vi "Query Deviation.vi"(8 "error in (no error)":errorcluster, 10 "Deviation Mode (0: Reading)":u16(ring) items=["Reading", "Absolute"], 11 "VISA resource name":refnum<visa-resource-name>) -> (0 "error out":errorcluster, 2 "Deviation":dbl format="%#_10g", 3 "VISA resource name out":refnum<visa-resource-name>)   [LabVIEW 2011, in "Fluke 8508.lvlib"]
doc: "This VI queries the stored standard deviations for a block of readings.\n\nNOTE: The instrument must be in Averaging or Block N mode for correct results to be displayed (Refer to Configure Averaging.vi to set the mode)."
uses:
  Fluke 8508.lvlib
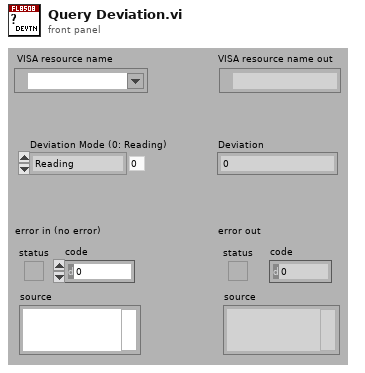
[diagram p1: front panel]
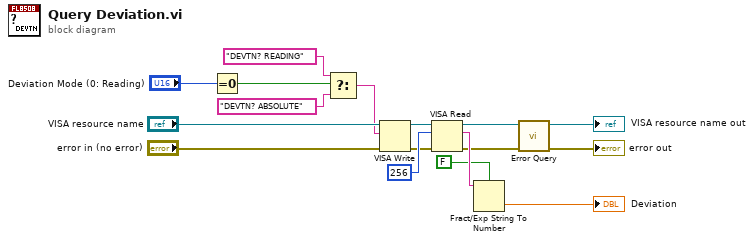
[diagram p0: block diagram]
diagram:
  n1 = Equal To 0?(x="Deviation Mode (0: Reading)") -> (x = 0?=w4:bool)
  n2 = Select(t="DEVTN? READING" ("write buffer"), s=w4, f="DEVTN? ABSOLUTE" ("write buffer")) -> (s? t:f=w5:string)
  n3 = VISA Write(VISA resource name="VISA resource name", write buffer=w5, error in (no error)="error in (no error)") -> (VISA resource name out=w16:refnum<visa-resource-name>, error out=w15:errorcluster)  [unwired: 1 out]
  n4 = VISA Read(VISA resource name=w16, byte count=u32 256, error in (no error)=w15) -> (VISA resource name out=w11:refnum<visa-resource-name>, read buffer=w14:string, error out=w10:errorcluster)  [unwired: 1 out]
  n5 = Fract/Exp String To Number(use system decimal point (T)=FALSE, string=w14) -> (number=→"Deviation":dbl)  [unwired: 2 in, 1 out]
  n6 = call "Error Query.vi"("error in (no error)"=w10, "VISA resource name"=w11) -> ("error out"=→"error out":errorcluster, "VISA resource name out"=→"VISA resource name out":refnum<visa-resource-name>)  [unwired: 6 in, 2 out]
